vi "get_amplitudes.vi"(0 "TrajectoryTS090820Circular2D in":refnum<class "TrajectoryTS090820Circular2D.lvclass">, 5 "error in (no error)":errorcluster) -> (14 "TrajectoryTS090820Circular2D out":refnum<class "TrajectoryTS090820Circular2D.lvclass">, 15 "x amplitude um":dbl[unit], 16 "y amplitude um":dbl[unit], 17 "x amplitude no units":dbl, 18 "y amplitude no units":dbl, 19 "error out":errorcluster)   [LabVIEW 2010, in "TrajectoryTS090820Circular2D.lvclass"]
uses:
  TrajectoryTS090820Circular2D.lvclass
  TrajectoryTS090820Circular2D.lvclass/TrajectoryTS090820Circular2D.ctl
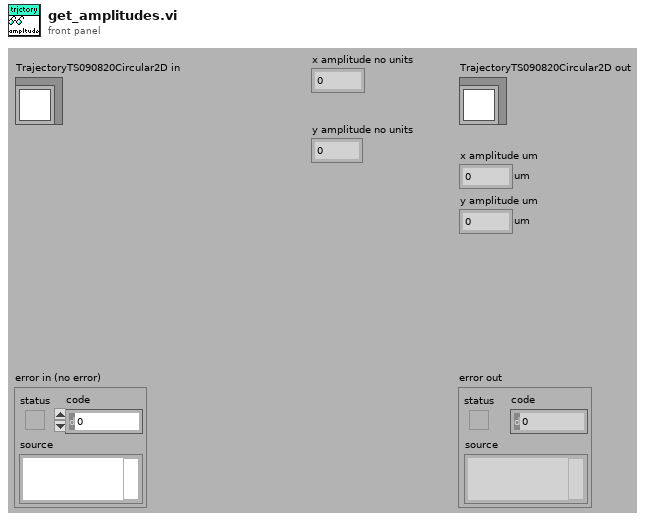
[diagram p1: front panel]
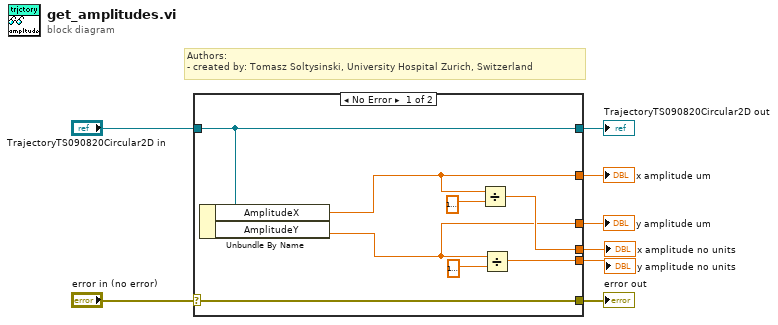
[diagram p0: block diagram]
diagram:
  # "Authors: \n- created by: Tomasz Soltysinski, University Hospital Zurich, Switzerland"
  n1 = case shown="No Error" "error in (no error)" {
    selector: "error in (no error)" -> [w16 w17]
    tunnel: [w16 w17] -> w7
    tunnel: [w15 w18] -> w5
    tunnel: "TrajectoryTS090820Circular2D in" -> [w15 w18]
    tunnel: [w10 _] -> w4
    tunnel: [w9 _] -> w3
    tunnel: [w12 _] -> w2
    tunnel: [w11 _] -> w1
    frame No Error {
      n2 = Unbundle By Name(w15) -> ("AmplitudeX"=w10:dbl[unit], "AmplitudeY"=w9:dbl[unit])
      n3 = Divide(x=w10, y=dbl[unit] 1e-06 ("dimension size")) -> (x/y=w12:dbl)
      n4 = Divide(x=w9, y=dbl[unit] 1e-06 ("dimension size")) -> (x/y=w11:dbl)
    }
    frame Error {
    }
  }
  "error out" <- w7
  "TrajectoryTS090820Circular2D out" <- w5
  "x amplitude um" <- w4
  "y amplitude um" <- w3
  "x amplitude no units" <- w2
  "y amplitude no units" <- w1
